vi "FingerTaskHold.vi"() -> ()   [LabVIEW 2011]
doc: "This example is a template that gives the structure of a single-loop PID controller. This VI uses the PID Filter VI to reduce measurement noise. This VI also uses the PID Autotuning VI to tune the controller based on the closed-loop response. This VI also uses the Timed Loop to ensure deterministic execution.\n\nReplace the Dummy Input and Dummy Output VIs with code that communicates with a real-time target."
uses:
  <vilib>/addons/Digital Filter Design/_Objects.llb/DFD Filter Obj.ctl
  <vilib>/addons/Digital Filter Design/_Objects.llb/DFD Filter Coef.ctl
  <vilib>/addons/Digital Filter Design/_Objects.llb/DFD Filter Structure Type Selector.ctl
  <vilib>/addons/Digital Filter Design/_Objects.llb/dfd_Internal Quantization Settings.ctl
  <vilib>/addons/Digital Filter Design/_Objects.llb/dfd_Internal Quantization Srcs.ctl
  <vilib>/addons/Digital Filter Design/_Objects.llb/DFD Coef Norm Type.ctl
  <vilib>/Platform/TimedLoop/XDataNode/timing_clust.ctl
  <vilib>/Platform/TimedLoop/XDataNode/nitl_modes.ctl
  <vilib>/Platform/TimedLoop/XDataNode/wakeup.ctl
  <vilib>/DAQmx/write.llb/DAQmx Write (Counter Frequency 1Chan 1Samp).vi
  <vilib>/DAQmx/write.llb/DAQmx Write (Digital 1D Bool NChan 1Samp 1Line).vi
  <vilib>/DAQmx/read.llb/DAQmx Read (Counter DBL 1Chan 1Samp).vi
  <vilib>/DAQmx/read.llb/DAQmx Read (Analog 1D DBL NChan 1Samp).vi
  <vilib>/addons/control/pid/pid.llb/PID Advanced (DBL Array).vi
  <vilib>/DAQmx/write.llb/DAQmx Write (Analog DBL 1Chan 1Samp).vi
  <vilib>/DAQmx/write.llb/DAQmx Write (Analog 1D DBL NChan 1Samp).vi
  <vilib>/addons/control/pid/pid.llb/PID Derivative Action Buffered (DBL Array).vi
  <vilib>/addons/control/pid/pid.llb/PID Get Advanced Error (DBL Array).vi
  <vilib>/addons/control/pid/pid.llb/PID Integral Action Buffered (DBL Array).vi
  <vilib>/addons/control/pid/pid.llb/PID Resize 1D Array.vi
  <vilib>/addons/control/pid/pid.llb/PID Get Advanced Error (DBL).vi
  <vilib>/DAQmx/create/channels.llb/DAQmx Create Channel (CO-Pulse Generation-Frequency).vi
  <vilib>/DAQmx/configure/timing.llb/DAQmx Timing (Implicit).vi
  <vilib>/DAQmx/miscellaneous.llb/DAQmx Fill In Error Info.vi
  <vilib>/addons/Digital Filter Design/Process.llb/DFD Filtering (PtByPt NChan).vi
  <vilib>/addons/control/pid/pid.llb/PID Parameter Manager (DBL Array).vi
  <vilib>/Platform/TimedLoop/XDataNode/XDataNode.xnode
  <vilib>/Platform/TimedLoop/XDataNode/XDNodeRunTimeDep.lvlib
  <vilib>/addons/Digital Filter Design/NI_DigFilterLicensed.lvlib
  <vilib>/addons/control/pid/NI_PID_pid.lvlib
panel:
  out "LastCount":u64
  out "error out 2":errorcluster
  out "error out":errorcluster
  in  "Timing":T1={"JuiceTime"=1000.0, "AbortTime"=1000.0, "RampTime"=500, "HoldTime"=1000, "ASD"=500}
  in  "RecordsSelection":string(combo)
  in  "Database":T2={"ExperimentDate"=timestamp(3401556199.892892 s since 1904-01-01), "ImplantDate"=timestamp(3401890063 s since 1904-01-01), "CerebusFolder"="", "Experimenter"="Tyler Davis", "PatientNumber"="201102", "DominantHand"="Right", "DeviceType"="uECOG", "DeviceSerial"="CG-64BPX-F419", "DeviceHemisphere"="Right", "DeviceRegion"="Hand", "TaskType"="ArmMovementTask.vi", "TaskComments"="", "RecordingComments"="", "GeneralObservations"=""}
  in  "CerebusConfigFile":path=path "E:/Code/TaskAutomation/ConfigFiles/32ChanRecording2K.mat"
  out "DatabaseUDL":path=path "E:/Data/PatientDatabase.udl"
  out "DataFolder":string
  out "TaskType":string
  out "Recording":bool
  out "StartTime":timestamp
  in  "MaxForce":dbl
  out "Middle":dbl(slide)=4.88375 scale=0.0..6.0
  out "Index":dbl(slide)=4.76025 scale=0.0..6.0
  out "Thumb":dbl(slide)=4.62875 scale=0.0..6.0
  in  "RandForce":bool
  in  "RampGain":dbl[](array[numeric])=[3.0, 3.0, 3.0] caption="Ramp Force"
  out "EncStartPos":cluster{"Index":dbl, "Middle":dbl, "Ring":dbl}={"Index"=3.1270000000000002, "Middle"=3.3110000000000004, "Ring"=3.0875000000000004}
  in  "HoldRange":dbl[](array[numeric])=[1.0, 1.0, 1.0]
  in  "RandFinger":bool=TRUE
  in  "InitialForce":dbl[](array[numeric])=[1.0, 1.0, 1.0] min=-10.0 max=10.0 step=1.0
  out "SlowLoop":bool
  out "SetPtOut":cluster{"[0]":dbl, "[1]":dbl, "[2]":dbl}(graph)={"[0]"=-0.023249999999999993, "[1]"=-0.6442500000000004, "[2]"=0.49950000000000294} caption="Set Point"
  out "LoadCell":cluster{"[0]":dbl, "[1]":dbl, "[2]":dbl}(graph)={"[0]"=-0.06598031273279871, "[1]"=-0.6487244867483078, "[2]"=0.44124715755068283} caption="Force"
  out "LoopPeriod":u64=10
  in  "DesiredPos":dbl[](array[numeric])=[3.0, 3.0, 3.0]
  out "EncPos":cluster{"[0]":dbl, "[1]":dbl, "[2]":dbl}(graph)={"[0]"=4.76025, "[1]"=4.88375, "[2]"=4.62875} caption="Position"
  out "TrialType":i32=1
  out "TrialCount":i32=2
  out "LoopCount":u64=1552
  out "Current State":T3(ring)=enum."Acquire Start"
  out "Finalize":enum16{"Reward", "Cerebus", "Reset"}(ring)
  out "Outcome":string="--"
  in  "Linearity":dbl=1.0 format="%.2f"
  out "PIDGainsOut":T4(array[cluster])=[{"proportional gain (Kc)"=0.4600000000000001, "integral time (Ti, min)"=0.0, "derivative time (Td, min)"=0.0}, {"proportional gain (Kc)"=0.4600000000000001, "integral time (Ti, min)"=0.0, "derivative time (Td, min)"=0.0}, {"proportional gain (Kc)"=0.4600000000000001, "integral time (Ti, min)"=0.0, "derivative time (Td, min)"=0.0}]
  in  "PIDGains":T5={"proportional high (Kc)"=0.5, "integral high (Ti, min)"=0.0, "derivative high (Td, min)"=0.0, "derivative low (Td, min)"=0.0, "integral low (Ti, min)"=0.0, "proportional low (Kc)"=0.1} caption="PID Gains"
  in  "PWMFreq(Hz)":dbl=20000.0 caption="PWM (Hz)" format="%#.6f"
  out "EncMax":dbl[](array[numeric])=[6.508000000000001, 6.507000000000001, 6.469500000000001]
  in  "BndrsCluster":T6={"InwardLimit(%)"=[0.7, 0.7, 0.7], "OutwardLimit(%)"=[0.3, 0.3, 0.3], "SpringCnst"=[5.0, 5.0, 5.0]} caption="Boundaries"
  out "LP_LoadCell":T7={"mSRate_Fs"=500.0, "mSRate_Version"="2.0", "mSRate_Comments"="", "mSRate_OrgCoef"={"type"=enum."IIR Cascaded Second Order Sections Form II Transposed", "gain"=1.0, "coef a (k)"=[-0.36952737735124136, 0.1958157126558331], "coef b (v)"=[0.20657208382614797, 0.41314416765229595, 0.20657208382614797]}, "mSRate_CurCoef"={"type"=enum."IIR Cascaded Second Order Sections Form II Transposed", "gain"=1.0, "coef a (k)"=[-0.36952737735124136, 0.1958157126558331], "coef b (v)"=[0.20657208382614797, 0.41314416765229595, 0.20657208382614797]}, "mSRate_Quantized?"=FALSE, "mSRate_QCoef"={"type"=enum."Undefined", "gain"=1.0, "coef a (k)"=[], "coef b (v)"=[]}, "mSRate_QSettings"=[], "mSRate_Order"=2, "mSRate_Scaling"={"mSRate_ScaleByPowerOf2?"=FALSE, "mSRate_ScaleType"=enum."No Norm"}} {"mSRate_QSettings"."source" items=["Coef a/k"=0, "Coef b/v"=7, "Input"=1, "Output"=2, "Multiplicand"=3, "Product"=4, "Sum"=5, "Delay"=6, "Gain"=8]}
  in  "LP_LoadCell(Hz)":dbl=100.0
  out "MotorDir":bool[](array[boolean])=[TRUE, TRUE, TRUE]
  in  "LoopFreq(Hz)":dbl=500.0 caption="Loop Period (us)"
  out "SetPoint":dbl[](array[numeric])=[1.0, 1.0, 1.0] caption="Set Point" min=-10.0 max=10.0 step=1.0
  out "PWMTaskC":refnum<k21>
  out "PWMTaskB":refnum<k21>
  in  "PIDLimit":dbl=0.5 caption="MaxDutyCycle" min=0.0 max=1.0 step=0.01 format="%.2f"
  out "LoopPeriodPID(s)":dbl=0.002 caption="Loop Period PID (s)" format="%#_10g"
  out "PWMTaskA":refnum<k21>
  out "LoopDuration(us)":i64=965 caption="Actual Loop Period (us)"
  in  "Stop":bool
  out "SlowLoopPID":bool
  # "index"
  # "middle"
  # "thumb"
  # "limits = -10 to 10 lbs"
  # "limits = 0 to 6 in"
  # "all time in ms"
  # "Do not place ';' or '=' in the comment fields"
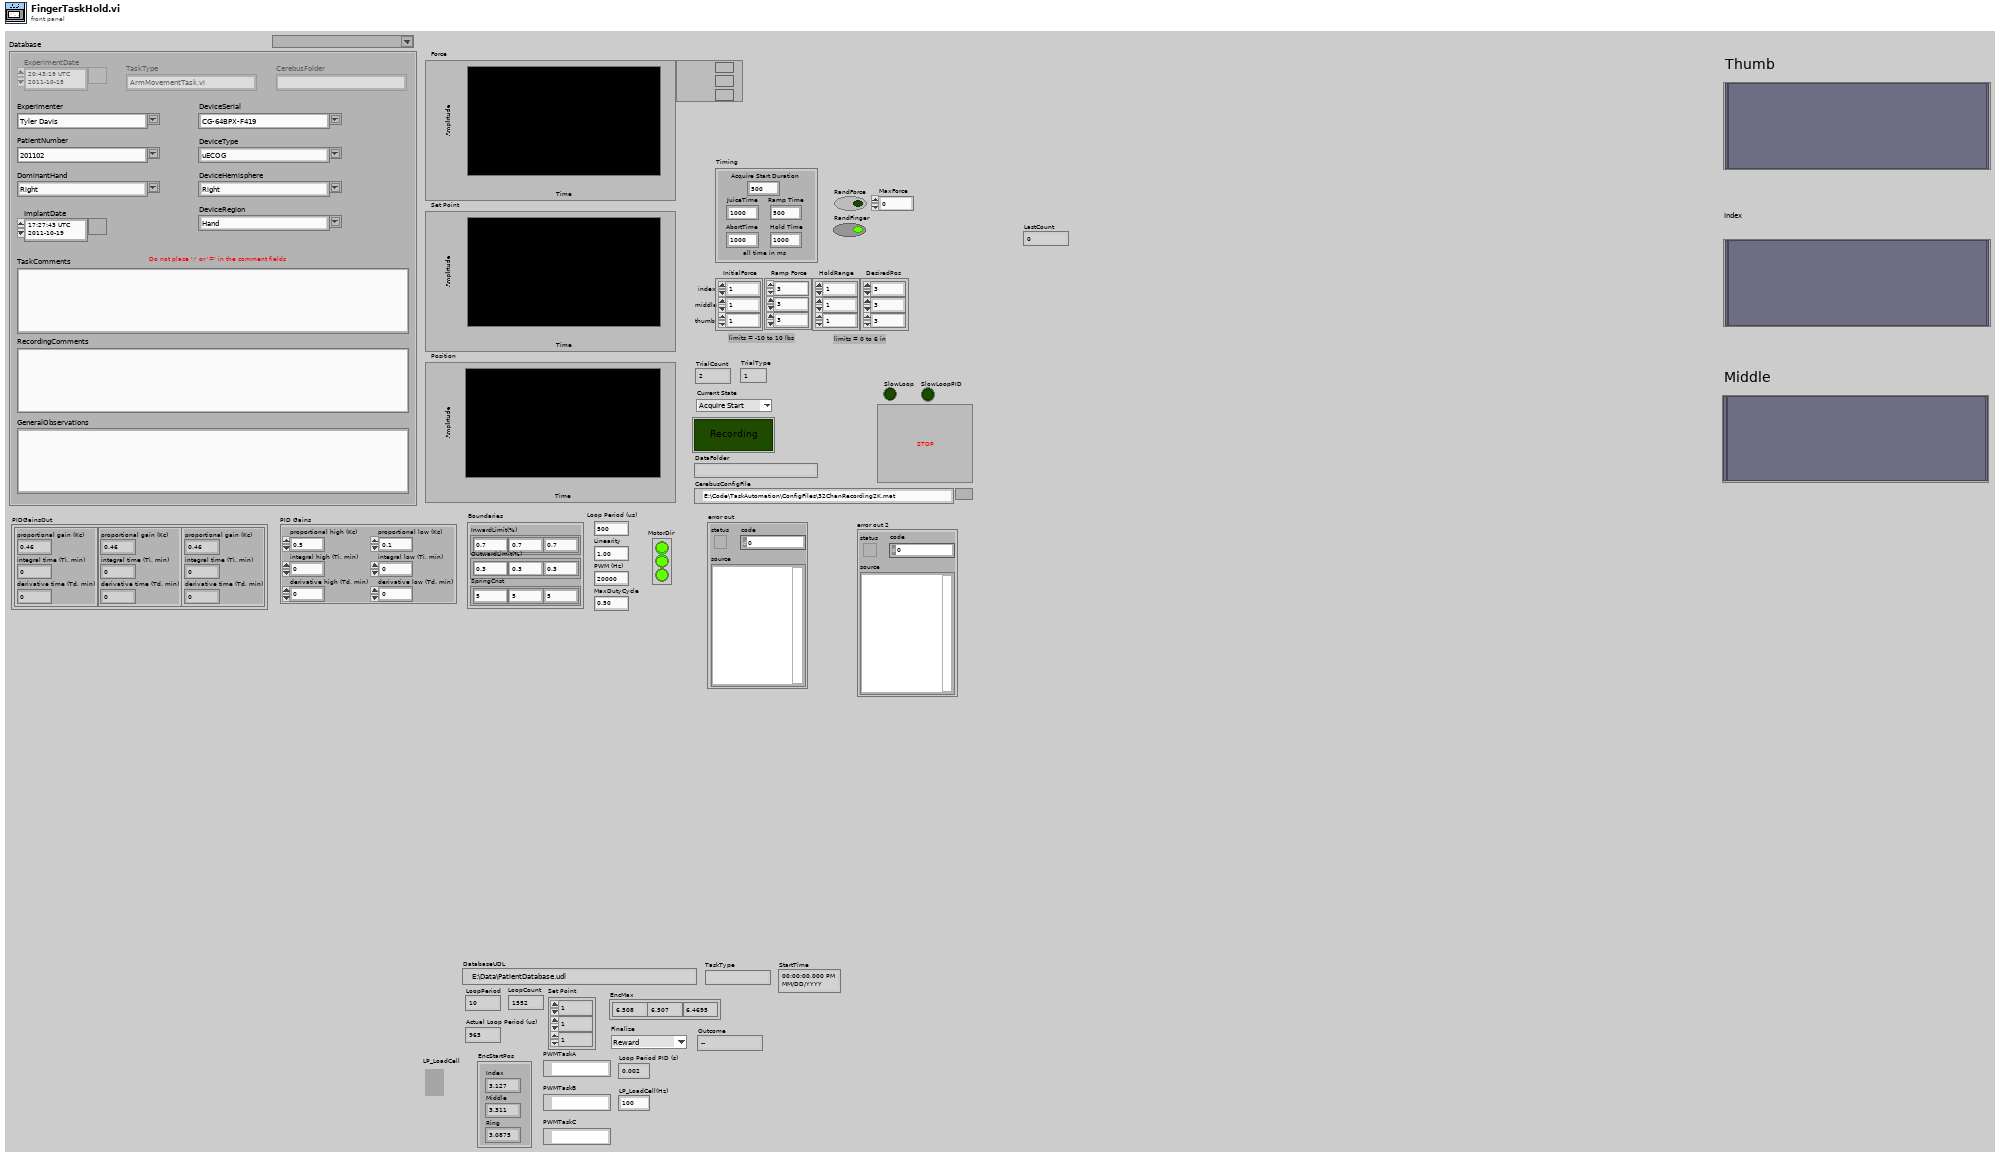
[diagram p1: front panel]
types:
  T1 = cluster{"JuiceTime":dbl, "AbortTime":dbl, "RampTime":u64, "HoldTime":u64, "ASD":u64}
  T2 = cluster{"ExperimentDate":timestamp, "ImplantDate":timestamp, "CerebusFolder":string, "Experimenter":string, "PatientNumber":string, "DominantHand":string, "DeviceType":string, "DeviceSerial":string, "DeviceHemisphere":string, "DeviceRegion":string, "TaskType":string, "TaskComments":string, "RecordingComments":string, "GeneralObservations":string}
  T3 = enum16{"Initialize", "Acquire Start", "Acquire Response", "Finalize"}
  T4 = cluster{"proportional gain (Kc)":dbl, "integral time (Ti, min)":dbl, "derivative time (Td, min)":dbl}[]
  T5 = cluster{"proportional high (Kc)":dbl, "integral high (Ti, min)":dbl, "derivative high (Td, min)":dbl, "derivative low (Td, min)":dbl, "integral low (Ti, min)":dbl, "proportional low (Kc)":dbl}
  T6 = cluster{"InwardLimit(%)":dbl[], "OutwardLimit(%)":dbl[], "SpringCnst":dbl[]}
  T7 = typedef "NI_DigFilterLicensed.lvlib/DFD Filter Obj.ctl" = cluster{"mSRate_Fs":dbl, "mSRate_Version":string, "mSRate_Comments":string, "mSRate_OrgCoef":T8, "mSRate_CurCoef":T8, "mSRate_Quantized?":bool, "mSRate_QCoef":T8, "mSRate_QSettings":T10[], "mSRate_Order":i32, "mSRate_Scaling":cluster{"mSRate_ScaleByPowerOf2?":bool, "mSRate_ScaleType":T12}}
  T8 = typedef "NI_DigFilterLicensed.lvlib/DFD Filter Coef.ctl" = cluster{"type":T9, "gain":dbl, "coef a (k)":dbl[], "coef b (v)":dbl[]}
  T9 = typedef "NI_DigFilterLicensed.lvlib/DFD Filter Structure Type Selector.ctl" = enum16{"Undefined", "FIR Direct Form", "FIR Direct Form Transposed", "FIR Symmetric", "FIR Antisymmetric", "IIR Direct Form I", "IIR Direct Form I Transposed", "IIR Direct Form II", "IIR Direct Form II Transposed", "IIR Cascaded Second Order Sections Form I", "IIR Cascaded Second Order Sections Form I Transposed", "IIR Cascaded Second Order Sections Form II", "IIR Cascaded Second Order Sections Form II Transposed", "Lattice Allpass (basic sections)", "Lattice Allpass (one multiplier sections)", "Lattice Allpass (normalized sections)", "Lattice AR (basic sections)", "Lattice AR (one multiplier sections)", "Lattice AR (normalized sections)", "Lattice MA (minimum phase)", "Lattice MA (maximum phase)", "Lattice ARMA (basic sections)", "Lattice ARMA (one multiplier sections)", "Lattice ARMA (normalized sections)"}
  T10 = typedef "NI_DigFilterLicensed.lvlib/dfd_Internal Quantization Settings.ctl" = cluster{"source":T11, "wl":i16, "iwl":i16, "overflow mode":enum16{"Saturation", "Wrap"}, "rounding mode":enum16{"Nearest", "Truncation"}, "signed?":bool}
  T11 = typedef "NI_DigFilterLicensed.lvlib/dfd_Internal Quantization Srcs.ctl" = u16
  T12 = typedef "NI_DigFilterLicensed.lvlib/DFD Coef Norm Type.ctl" = enum16{"No Norm", "Time Domain 1-Norm", "Time Domain 2-Norm", "Time Domain Inf-Norm"}
  T13 = enum16{"Initialize", "String", "Start", "New Session", "Stop", "Resume", "Close"}
  T14 = enum16{"SaveConfiguration", "StartRecording", "StopRecording"}
  T15 = typedef "XDNodeRunTimeDep.lvlib/timing_clust.ctl" = cluster{"Expected End [f-1]":u64, "Actual End [f-1]":u64, "Finished Late? [f-1]":bool, "Expected End [i-1]":u64, "Actual End [i-1]":u64, "Finished Late? [i-1]":bool, "Expected Start [i]":u64, "Actual Start [i]":u64, "Expected Start [f]":u64, "Actual Start [f]":u64, "Source Name":string, "Structure Name":string, "Period":i64, "Deadline":i64, "Offset":i64, "Start":i64, "Priority":i32, "Timeout":i32, "Mode":T16, "Wakeup Reason":T17, "Error":errorcluster, "Source Type":string, "Secondary Source Type":string, "Global End Time":u64, "Global Start Time":u64, "Frame Duration":u64, "Iteration Duration":u64, "Assigned CPU":i32, "I/O Scan Engine Mode":u32}
  T16 = typedef "XDNodeRunTimeDep.lvlib/nitl_modes.ctl" = enum32{"No Change", "Process missed periods, maintain original phase", "Discard missed periods, maintain original phase", "Process missed periods, ignore original phase", "Discard missed periods, ignore original phase"}
  T17 = typedef "XDNodeRunTimeDep.lvlib/wakeup.ctl" = enum32{"Normal", "Aborted", "Asynchronous wakeup", "Timing source error", "Timed loop error", "Timeout"}
  T18 = enum16{"Lowpass", "Highpass", "Bandpass", "Bandstop"}
  T19 = typedef "LVAllMonitorsDisplayTypeDef.ctl" = cluster{"Bounds":cluster{"Left":i16, "Top":i16, "Right":i16, "Bottom":i16}, "Depth":i16}[]
  T20 = cluster{"Disp.AllMonitors[0]":cluster{"Bounds":cluster{"Left":i16, "Top":i16, "Right":i16, "Bottom":i16}, "Depth":i16}, "Disp.AllMonitors[1]":cluster{"Bounds":cluster{"Left":i16, "Top":i16, "Right":i16, "Bottom":i16}, "Depth":i16}, "Disp.AllMonitors[2]":cluster{"Bounds":cluster{"Left":i16, "Top":i16, "Right":i16, "Bottom":i16}, "Depth":i16}, "Disp.AllMonitors[3]":cluster{"Bounds":cluster{"Left":i16, "Top":i16, "Right":i16, "Bottom":i16}, "Depth":i16}, "Disp.AllMonitors[4]":cluster{"Bounds":cluster{"Left":i16, "Top":i16, "Right":i16, "Bottom":i16}, "Depth":i16}, "Disp.AllMonitors[5]":cluster{"Bounds":cluster{"Left":i16, "Top":i16, "Right":i16, "Bottom":i16}, "Depth":i16}, "Disp.AllMonitors[6]":cluster{"Bounds":cluster{"Left":i16, "Top":i16, "Right":i16, "Bottom":i16}, "Depth":i16}, "Disp.AllMonitors[7]":cluster{"Bounds":cluster{"Left":i16, "Top":i16, "Right":i16, "Bottom":i16}, "Depth":i16}, "Disp.AllMonitors[8]":cluster{"Bounds":cluster{"Left":i16, "Top":i16, "Right":i16, "Bottom":i16}, "Depth":i16}}
  T21 = cluster{"Left":i16, "Top":i16, "Right":i16, "Bottom":i16}
  T22 = cluster{"Left":bool, "Top":bool, "Right":bool, "Bottom":bool}
  T23 = typedef "LVRectTypeDef.ctl" = cluster{"left":i16, "top":i16, "right":i16, "bottom":i16}
  T24 = typedef "LVPointTypeDef.ctl" = cluster{"Horizontal":i16, "Vertical":i16}
  T25 = cluster{"SetPointOut[0]":dbl, "SetPointOut[1]":dbl, "SetPointOut[2]":dbl}
  T26 = cluster{"signal out[0]":dbl, "signal out[1]":dbl, "signal out[2]":dbl}
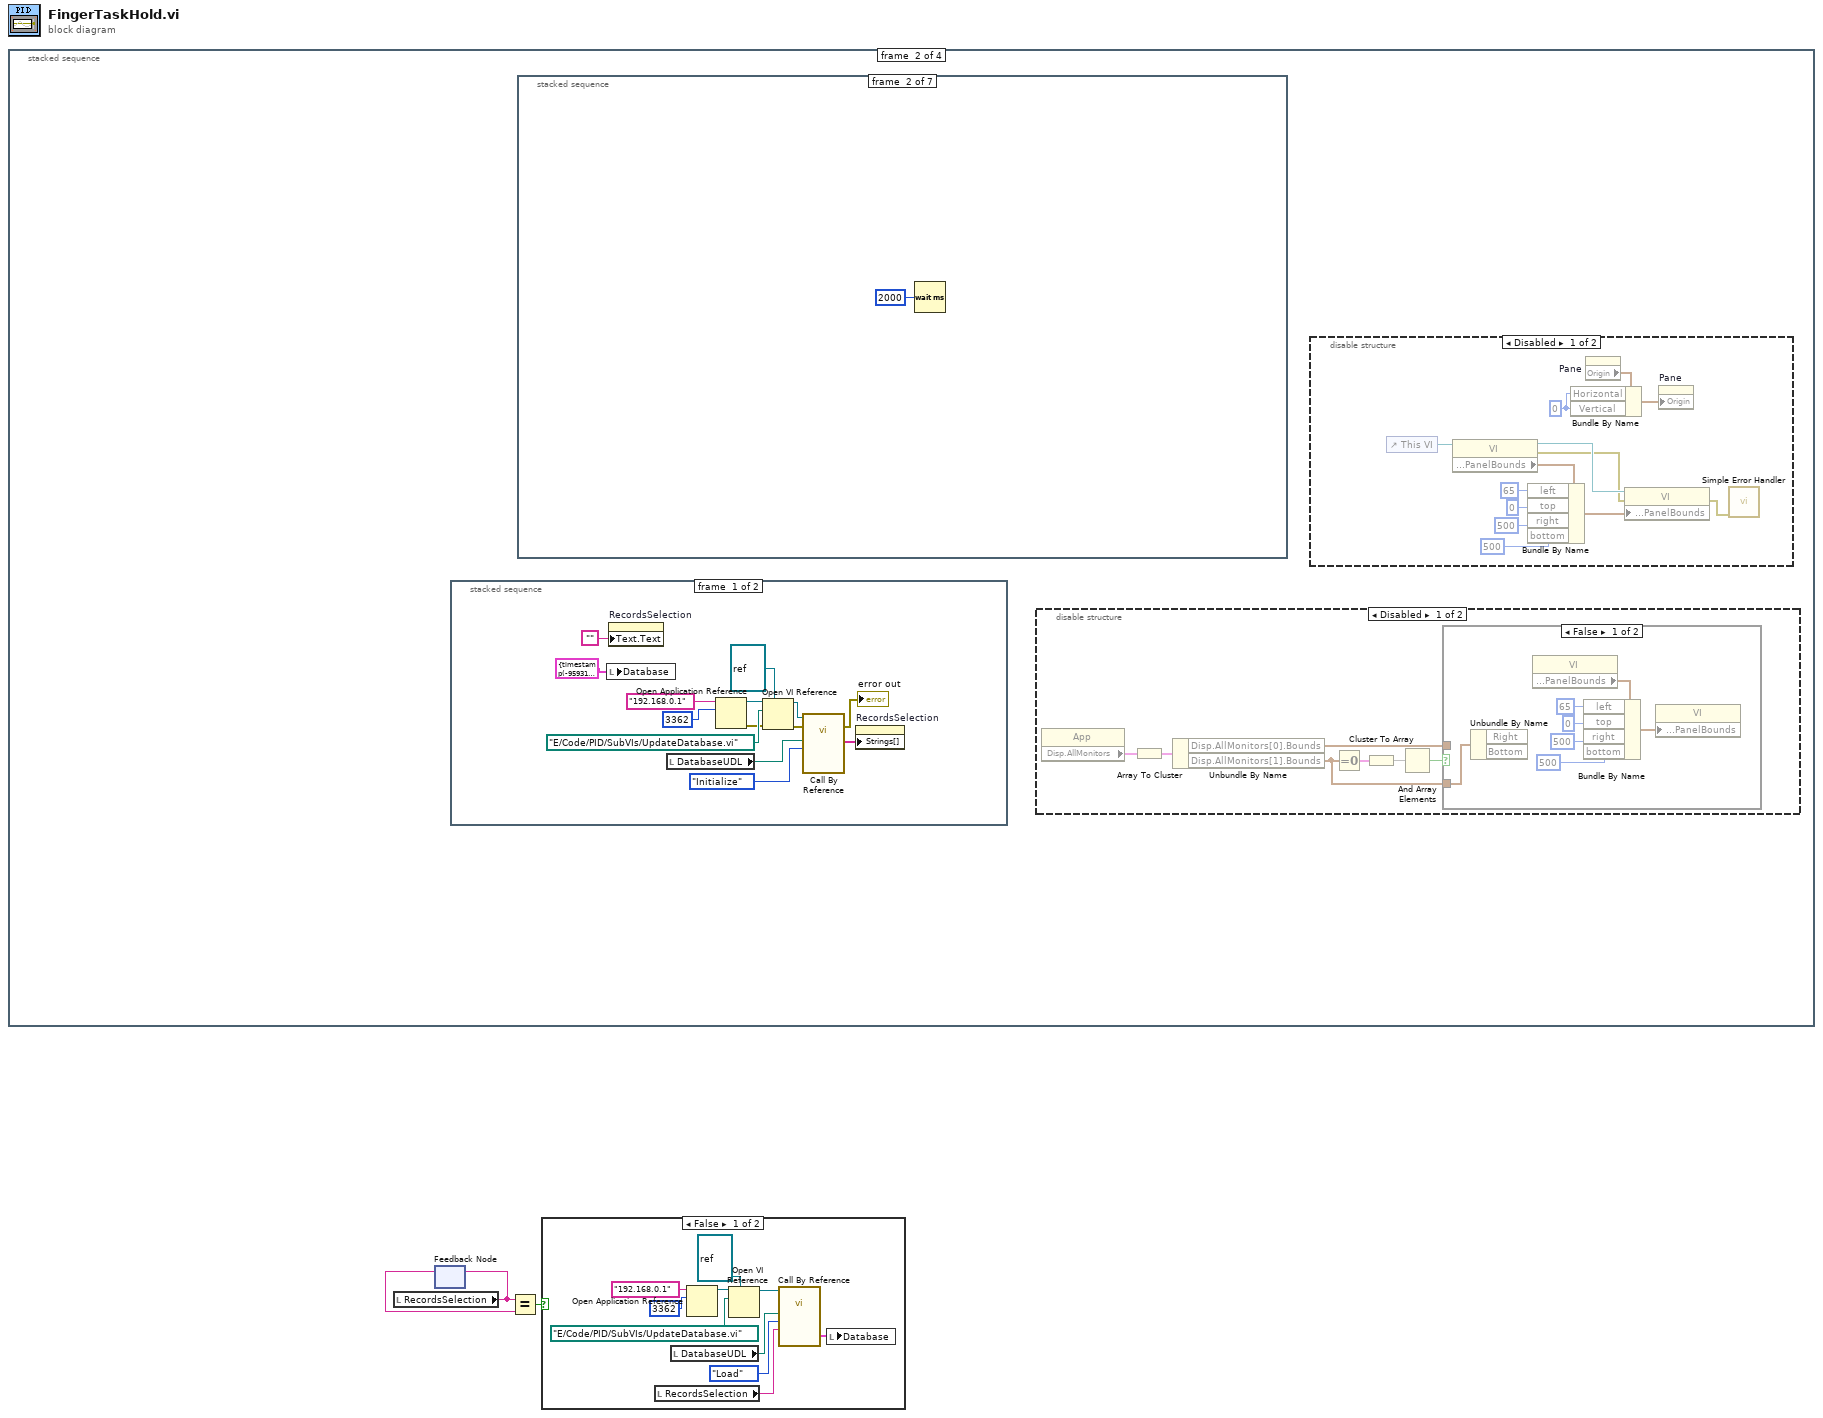
[diagram p0: block diagram]
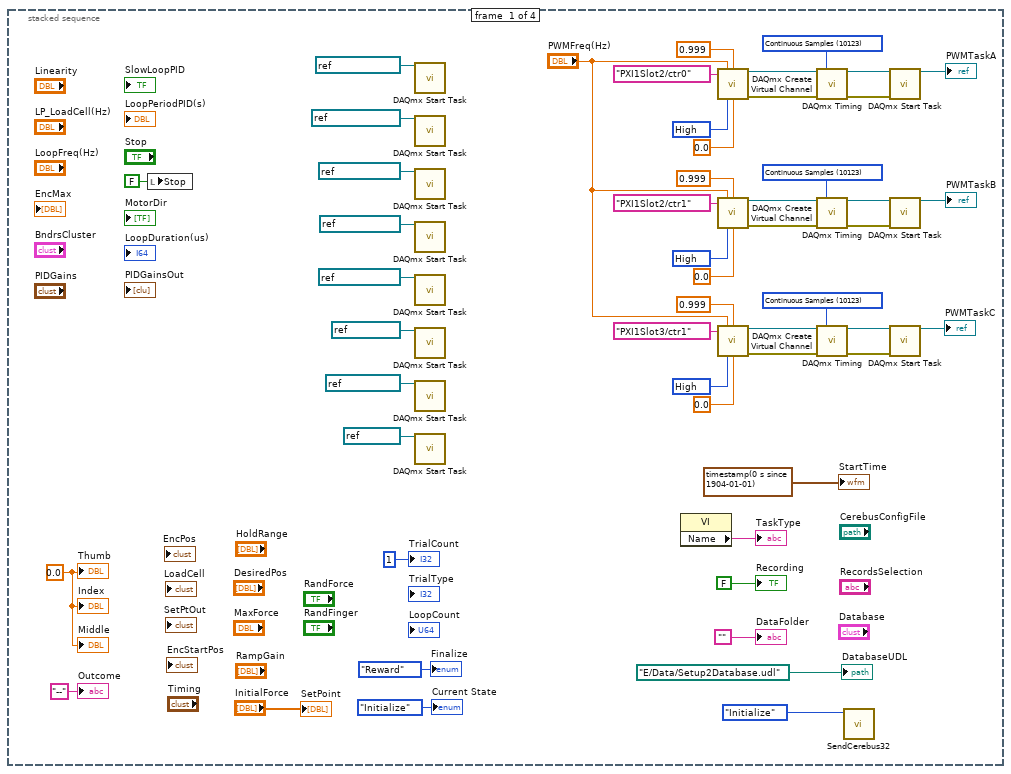
[diagram p3: hidden frame]
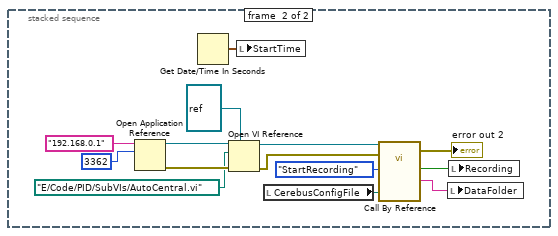
[diagram p4: hidden frame]
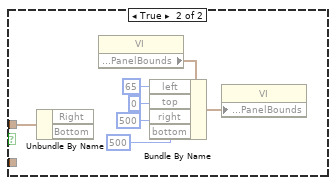
[diagram p6: hidden frame]
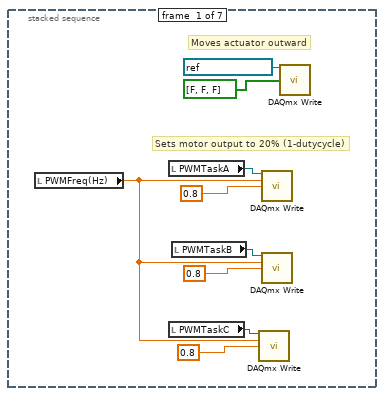
[diagram p8: hidden frame]
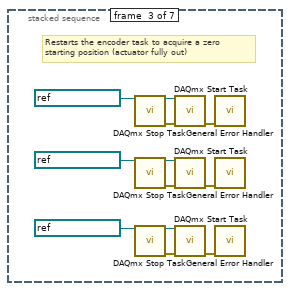
[diagram p9: hidden frame]
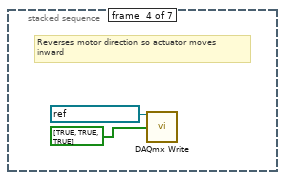
[diagram p10: hidden frame]
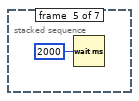
[diagram p11: hidden frame]
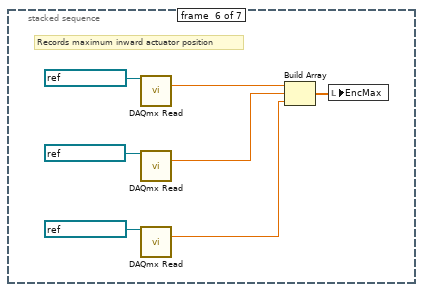
[diagram p12: hidden frame]
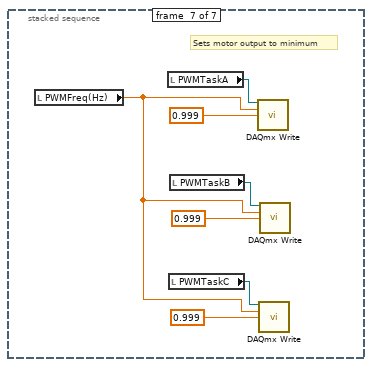
[diagram p13: hidden frame]
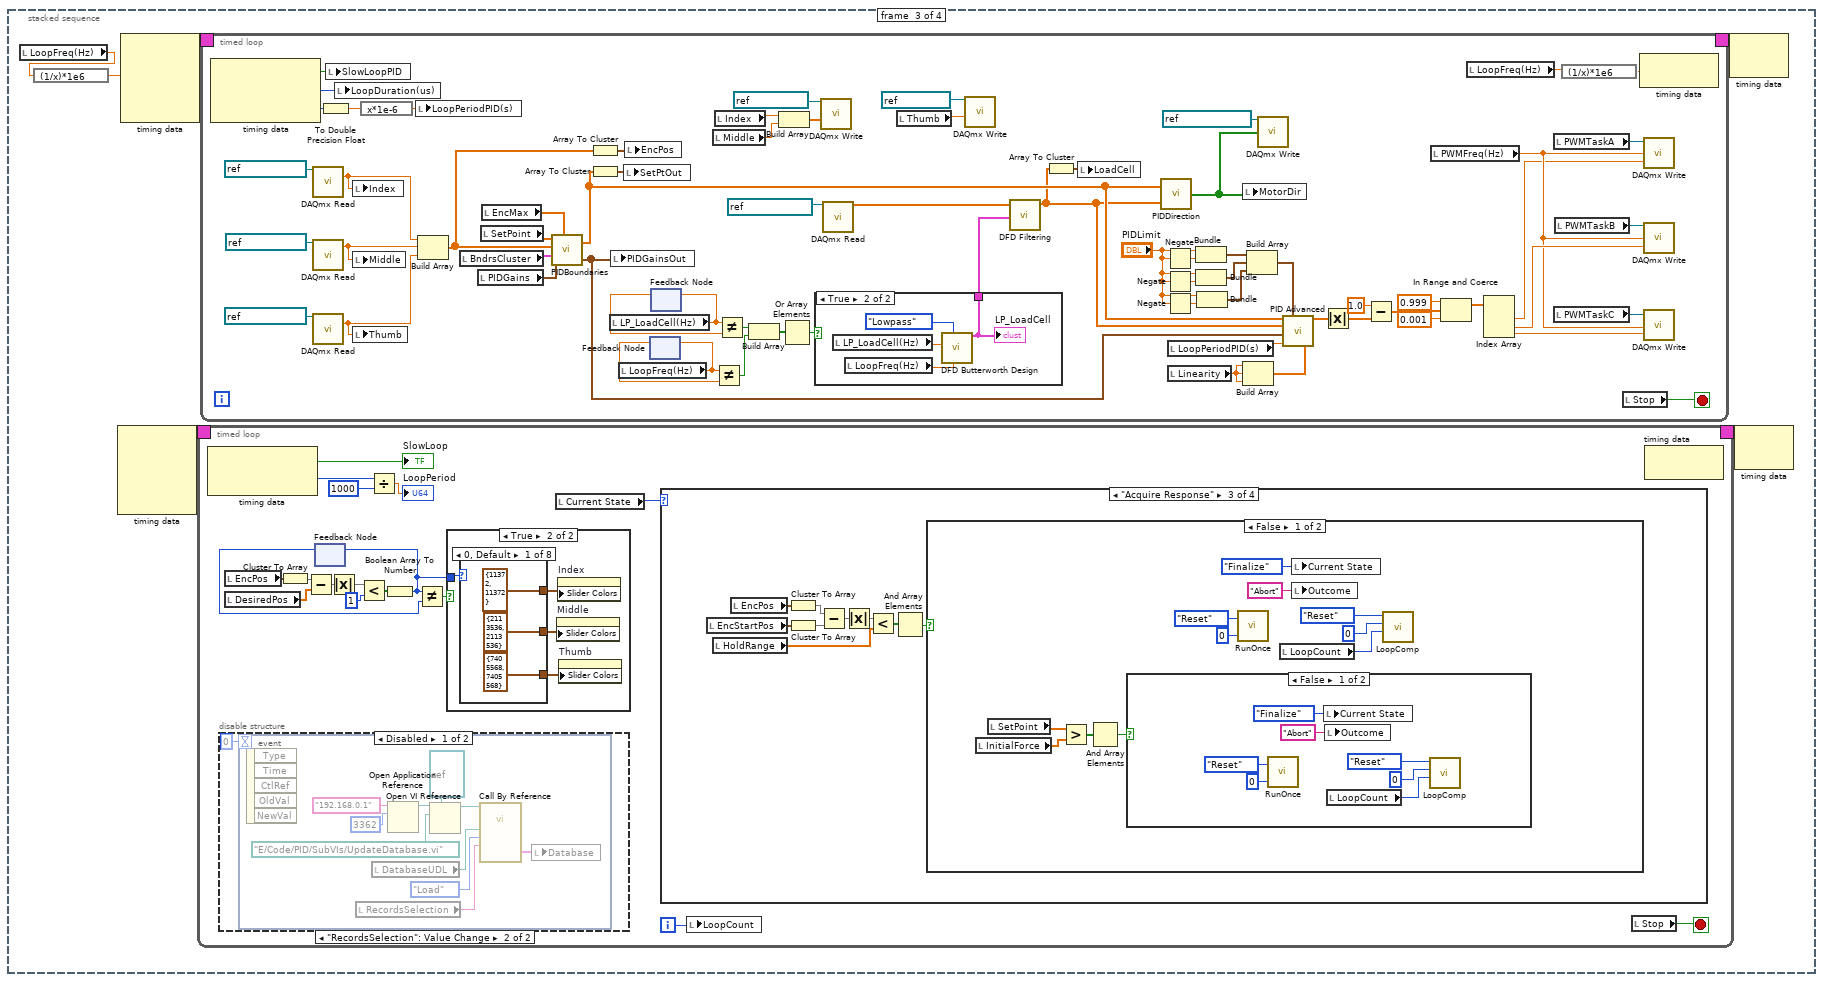
[diagram p14: hidden frame]
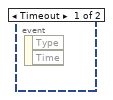
[diagram p15: hidden frame]
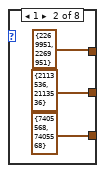
[diagram p18: hidden frame]
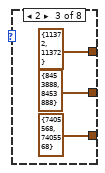
[diagram p19: hidden frame]
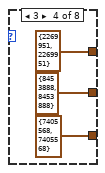
[diagram p20: hidden frame]
diagram:
  n1 = stacked-sequence {
    frame #0 {
      w11 = 0.0 ("THUMB")
      w28 = 10192 items=["High"=10192, "Low"=10214] ("idle state")
      w22 = 10123 items=["Finite Samples"=10178, "Continuous Samples"=10123] ("sample mode")
      w35 = 10192 items=["High"=10192, "Low"=10214] ("idle state")
      w41 = 10123 items=["Finite Samples"=10178, "Continuous Samples"=10123] ("sample mode")
      w52 = 10192 items=["High"=10192, "Low"=10214] ("idle state")
      w45 = 10123 items=["Finite Samples"=10178, "Continuous Samples"=10123] ("sample mode")
      n2 = local write "Stop"(FALSE ("stop")) -> ()
      n3 = call <vilib>:"DAQmx Start Task.vi"("task/channels in"=refnum<k21> "ForceInABC") -> ()  [unwired: 13 in, 2 out]
      n4 = call <vilib>:"DAQmx Start Task.vi"("task/channels in"=refnum<k21> "MotorDirABC") -> ()  [unwired: 13 in, 2 out]
      n5 = call <vilib>:"DAQmx Start Task.vi"("task/channels in"=refnum<k21> "PositionInA") -> ()  [unwired: 13 in, 2 out]
      n6 = call <vilib>:"DAQmx Start Task.vi"("task/channels in"=refnum<k21> "PositionInB" ("task")) -> ()  [unwired: 13 in, 2 out]
      n7 = call <vilib>:"DAQmx Start Task.vi"("task/channels in"=refnum<k21> "PositionInC") -> ()  [unwired: 13 in, 2 out]
      n8 = call <vilib>:"DAQmx Start Task.vi"("task/channels in"=refnum<k21> "PosOutT" ("task")) -> ()  [unwired: 13 in, 2 out]
      n9 = call <vilib>:"DAQmx Start Task.vi"("task/channels in"=refnum<k21> "PosOutIM") -> ()  [unwired: 13 in, 2 out]
      n10 = call <vilib>:"DAQmx Start Task.vi"("task/channels in"=refnum<k21> "sound") -> ()  [unwired: 13 in, 2 out]
      n11 = property class="VI"() -> ("Name"=→"TaskType":string)  [unwired: 2 in, 2 out]
      n12 = call-poly <vilib>:"DAQmx Create Virtual Channel.vi"("frequency"="PWMFreq(Hz)", "duty cycle"=0.999, "counter"=tag "PXI1Slot2/ctr0", "idle state"=w52, "initial delay"=0.0) -> ("task out"=w48:refnum<k21>, "error out"=w49:errorcluster)  [unwired: 9 in]
      n13 = call-poly <vilib>:"DAQmx Create Virtual Channel.vi"("frequency"="PWMFreq(Hz)", "duty cycle"=0.999, "counter"=tag "PXI1Slot2/ctr1", "idle state"=w35, "initial delay"=0.0) -> ("task out"=w38:refnum<k21>, "error out"=w37:errorcluster)  [unwired: 9 in]
      n14 = call-poly <vilib>:"DAQmx Create Virtual Channel.vi"("frequency"="PWMFreq(Hz)", "duty cycle"=0.999, "counter"=tag "PXI1Slot3/ctr1", "idle state"=w28, "initial delay"=0.0) -> ("task out"=w25:refnum<k21>, "error out"=w26:errorcluster)  [unwired: 9 in]
      n15 = call-poly <vilib>:"DAQmx Timing.vi"("task/channels in"=w48, "sample mode"=w45, "error in"=w49) -> ("task out"=w46:refnum<k21>, "error out"=w47:errorcluster)  [unwired: 11 in]
      n16 = call-poly <vilib>:"DAQmx Timing.vi"("task/channels in"=w38, "sample mode"=w41, "error in"=w37) -> ("task out"=w40:refnum<k21>, "error out"=w39:errorcluster)  [unwired: 11 in]
      n17 = call-poly <vilib>:"DAQmx Timing.vi"("task/channels in"=w25, "sample mode"=w22, "error in"=w26) -> ("task out"=w23:refnum<k21>, "error out"=w24:errorcluster)  [unwired: 11 in]
      n18 = call "SendCerebus32.vi"("Mode"=T13."Initialize") -> ()  [unwired: 4 in]
      n19 = call <vilib>:"DAQmx Start Task.vi"("task/channels in"=w46, "error in"=w47) -> ("task out"=→"PWMTaskA":refnum<k21>)  [unwired: 12 in, 1 out]
      n20 = call <vilib>:"DAQmx Start Task.vi"("task/channels in"=w40, "error in"=w39) -> ("task out"=→"PWMTaskB":refnum<k21>)  [unwired: 12 in, 1 out]
      n21 = call <vilib>:"DAQmx Start Task.vi"("task/channels in"=w23, "error in"=w24) -> ("task out"=→"PWMTaskC":refnum<k21>)  [unwired: 12 in, 1 out]
      "SetPoint" <- "InitialForce"
      "Outcome" <- "--" ("Outcome")
      "Current State" <- T3."Initialize" ("Current State")
      "Finalize" <- enum16{"Reward", "Cerebus", "Reset"}."Reward" ("Finalize")
      "TrialCount" <- 1 ("TrialCount")
      "Thumb" <- w11
      "Index" <- w11
      "Middle" <- w11
      "StartTime" <- timestamp(0 s since 1904-01-01)
      "Recording" <- FALSE ("Recording")
      "DatabaseUDL" <- path "E:/Data/Setup2Database.udl" ("DatabaseUDL")
      "DataFolder" <- ""
    }
    frame #1 {
      n22 = stacked-sequence {
        frame #0 {
          n23 = local write "Database"(T2 {"ExperimentDate"=timestamp(-9593179200 s since 1904-01-01), "ImplantDate"=timestamp(-9593179200 s since 1904-01-01), "CerebusFolder"="", "Experimenter"="", "PatientNumber"="", "DominantHand"="", "DeviceType"="", "DeviceSerial"="", "DeviceHemisphere"="", "DeviceRegion"="", "TaskType"="", "TaskComments"="", "RecordingComments"="", "GeneralObservations"=""} ("Database")) -> ()
          n24 = property on="RecordsSelection" class="CmbBox"("Text.Text"="") -> ()  [unwired: 2 in, 2 out]
          n25 = local read "DatabaseUDL"() -> (w60:path)
          n26 = Open Application Reference(10:u16 3362 ("port number or service name (3363)"), 11:"192.168.0.1" ("machine name (\"\":  open local reference)")) -> (0:w58:errorcluster, 3:w65:refnum<vi>)  [unwired: 2 in]
          n27 = Open VI Reference(type specifier VI Refnum (for type only)=refnum<vi> refnum, application reference (local)=w65, vi path=path "E:/Code/PID/SubVIs/UpdateDatabase.vi", error in (no error)=w58) -> (vi reference=w62:refnum<vi>, error out=w57:errorcluster)  [unwired: 2 in]
          n28 = call-by-ref "?"(reference=w62, error in=w57, "CallType"=enum16{"Initialize", "Save", "Load"}."Initialize", "DatabaseUDL"=w60) -> (error out=→"error out":errorcluster, "ExperimentDatesSorted"=w59:string[])  [unwired: 2 in, 3 out]
          n29 = property on="RecordsSelection" class="CmbBox"("Strings[]"=w59) -> ()  [unwired: 2 in, 2 out]
        }
        frame #1 {
          n30 = Open Application Reference(10:u16 3362 ("port number or service name (3363)"), 11:"192.168.0.1" ("machine name (\"\":  open local reference)")) -> (0:w73:errorcluster, 3:w80:refnum<vi>)  [unwired: 2 in]
          n31 = Get Date/Time In Seconds() -> (seconds since 1Jan1904=w83:timestamp)
          n32 = Open VI Reference(type specifier VI Refnum (for type only)=refnum<vi> refnum, application reference (local)=w80, vi path=path "E:/Code/PID/SubVIs/AutoCentral.vi", error in (no error)=w73) -> (vi reference=w78:refnum<vi>, error out=w72:errorcluster)  [unwired: 2 in]
          n33 = local write "StartTime"(w83) -> ()
          n34 = local read "CerebusConfigFile"() -> (w76:path)
          n35 = call-by-ref "?"(reference=w78, error in=w72, "ConfigurationFile"=w76, "Mode"=T14."StartRecording") -> (error out=→"error out 2":errorcluster, "DataFolder"=w74:string, "Recording?"=w75:bool)  [unwired: 1 in, 2 out]
          n36 = local write "DataFolder"(w74) -> ()
          n37 = local write "Recording"(w75) -> ()
        }
      }
      n38 = stacked-sequence {
        frame #0 {
          # "Sets motor output to 20% (1-dutycycle)"
          # "Moves actuator outward"
          n39 = local read "PWMFreq(Hz)"() -> (w118:dbl)
          n40 = local read "PWMTaskA"() -> (w125:refnum<k21>)
          n41 = local read "PWMTaskC"() -> (w119:refnum<k21>)
          n42 = local read "PWMTaskB"() -> (w122:refnum<k21>)
          n43 = call-poly <vilib>:"DAQmx Write.vi"("task/channels in"=w119, "frequency"=w118, "duty cycle"=0.8) -> ()  [unwired: 10 in, 3 out]
          n44 = call-poly <vilib>:"DAQmx Write.vi"("task/channels in"=w125, "frequency"=w118, "duty cycle"=0.8) -> ()  [unwired: 10 in, 3 out]
          n45 = call-poly <vilib>:"DAQmx Write.vi"("task/channels in"=w122, "frequency"=w118, "duty cycle"=0.8) -> ()  [unwired: 10 in, 3 out]
          n46 = call-poly <vilib>:"DAQmx Write.vi"("task/channels in"=refnum<k21> "MotorDirABC", "data"=bool[] [FALSE, FALSE, FALSE]) -> ()  [unwired: 11 in, 3 out]
        }
        frame #1 {
          n47 = Wait (ms)(milliseconds to wait=u32 2000) -> ()  [unwired: 1 out]
        }
        frame #2 {
          # "Restarts the encoder task to acquire a zero\nstarting position (actuator fully out)"
          n48 = call <vilib>:"DAQmx Stop Task.vi"("task/channels in"=refnum<k21> "PositionInA") -> ("task out"=w137:refnum<k21>, "error out"=w136:errorcluster)  [unwired: 13 in]
          n49 = call <vilib>:"DAQmx Stop Task.vi"("task/channels in"=refnum<k21> "PositionInB") -> ("task out"=w134:refnum<k21>, "error out"=w135:errorcluster)  [unwired: 13 in]
          n50 = call <vilib>:"DAQmx Stop Task.vi"("task/channels in"=refnum<k21> "PositionInC") -> ("task out"=w129:refnum<k21>, "error out"=w128:errorcluster)  [unwired: 13 in]
          n51 = call <vilib>:"DAQmx Start Task.vi"("task/channels in"=w137, "error in"=w136) -> ("error out"=w139:errorcluster)  [unwired: 12 in, 1 out]
          n52 = call <vilib>:"DAQmx Start Task.vi"("task/channels in"=w134, "error in"=w135) -> ("error out"=w132:errorcluster)  [unwired: 12 in, 1 out]
          n53 = call <vilib>:"DAQmx Start Task.vi"("task/channels in"=w129, "error in"=w128) -> ("error out"=w131:errorcluster)  [unwired: 12 in, 1 out]
          n54 = call <vilib>:"General Error Handler.vi"("error in (no error)"=w139) -> ()  [unwired: 10 in, 5 out]
          n55 = call <vilib>:"General Error Handler.vi"("error in (no error)"=w132) -> ()  [unwired: 10 in, 5 out]
          n56 = call <vilib>:"General Error Handler.vi"("error in (no error)"=w131) -> ()  [unwired: 10 in, 5 out]
        }
        frame #3 {
          # "Reverses motor direction so actuator moves\ninward"
          n57 = call-poly <vilib>:"DAQmx Write.vi"("task/channels in"=refnum<k21> "MotorDirABC", "data"=bool[] [TRUE, TRUE, TRUE]) -> ()  [unwired: 11 in, 3 out]
        }
        frame #4 {
          n58 = Wait (ms)(milliseconds to wait=u32 2000) -> ()  [unwired: 1 out]
        }
        frame #5 {
          # "Records maximum inward actuator position"
          n59 = call-poly <vilib>:"DAQmx Read.vi"("task/channels in"=refnum<k21> "PositionInA") -> ("data"=w146:dbl)  [unwired: 12 in, 2 out]
          n60 = call-poly <vilib>:"DAQmx Read.vi"("task/channels in"=refnum<k21> "PositionInB") -> ("data"=w145:dbl)  [unwired: 12 in, 2 out]
          n61 = call-poly <vilib>:"DAQmx Read.vi"("task/channels in"=refnum<k21> "PositionInC") -> ("data"=w144:dbl)  [unwired: 12 in, 2 out]
          n62 = Build Array(w146, w145, w144) -> (w143:dbl[])
          n63 = local write "EncMax"(w143) -> ()
        }
        frame #6 {
          # "Sets motor output to minimum"
          n64 = local read "PWMFreq(Hz)"() -> (w150:dbl)
          n65 = local read "PWMTaskA"() -> (w155:refnum<k21>)
          n66 = local read "PWMTaskC"() -> (w151:refnum<k21>)
          n67 = local read "PWMTaskB"() -> (w154:refnum<k21>)
          n68 = call-poly <vilib>:"DAQmx Write.vi"("task/channels in"=w155, "frequency"=w150, "duty cycle"=0.999) -> ()  [unwired: 10 in, 3 out]
          n69 = call-poly <vilib>:"DAQmx Write.vi"("task/channels in"=w151, "frequency"=w150, "duty cycle"=0.999) -> ()  [unwired: 10 in, 3 out]
          n70 = call-poly <vilib>:"DAQmx Write.vi"("task/channels in"=w154, "frequency"=w150, "duty cycle"=0.999) -> ()  [unwired: 10 in, 3 out]
        }
      }
      n71 = disable-structure shown="Disabled" {
        frame Disabled {
          n72 = property class="App"() -> ("Disp.AllMonitors"=w97:T19)  [unwired: 2 in, 2 out]
          n73 = Array To Cluster(array=w97) -> (cluster=w98:T20)
          n74 = Unbundle By Name(w98) -> ("Disp.AllMonitors[0].Bounds"=w102:T21, "Disp.AllMonitors[1].Bounds"=w103:T21)
          n75 = Equal To 0?(x=w103) -> (x = 0?=w99:T22)
          n76 = Cluster To Array(cluster=w99) -> (array=w100:bool[])
          n77 = And Array Elements(Boolean array=w100) -> (logical AND=w101:bool)
          n78 = case shown="False" w101 {
            tunnel: w102 -> [_ w113]
            tunnel: w103 -> [w106 _]
            frame False {
              n79 = Unbundle By Name(w106) -> ()  [unwired: 2 out]
              n80 = property class="VI"() -> ("Front Panel.PanelBounds"=w107:T23)  [unwired: 2 in, 2 out]
              n81 = Bundle By Name(cluster=w107, "left"=i16 65, "top"=i16 0, "right"=i16 500, "bottom"=i16 500) -> (w108:T23)
              n82 = property class="VI"("Front Panel.PanelBounds"=w108) -> ()  [unwired: 2 in, 2 out]
            }
            frame True {
              n83 = Unbundle By Name(w113) -> ()  [unwired: 2 out]
              n84 = property class="VI"() -> ("Front Panel.PanelBounds"=w114:T23)  [unwired: 2 in, 2 out]
              n85 = Bundle By Name(cluster=w114, "left"=i16 65, "top"=i16 0, "right"=i16 500, "bottom"=i16 500) -> (w115:T23)
              n86 = property class="VI"("Front Panel.PanelBounds"=w115) -> ()  [unwired: 2 in, 2 out]
            }
          }
        }
        frame Enabled {
        }
      }
      n87 = disable-structure shown="Disabled" {
        frame Disabled {
          w96 = i16 0 ("Vertical")
          n88 = control-ref of="This VI"() -> (w85:refnum<vi>)
          n89 = property class="VI"(reference=w85) -> (reference out=w87:refnum<vi>, error out=w84:errorcluster, "Front Panel.PanelBounds"=w91:T23)  [unwired: 1 in]
          n90 = Bundle By Name(cluster=w91, "left"=i16 65, "top"=i16 0, "right"=i16 500, "bottom"=i16 500) -> (w90:T23)
          n91 = property on="Pane" class="Pane"() -> ("Origin"=w95:T24)  [unwired: 2 in, 2 out]
          n92 = Bundle By Name(cluster=w95, "Horizontal"=w96, "Vertical"=w96) -> (w94:T24)
          n93 = property class="VI"(reference=w87, error in=w84, "Front Panel.PanelBounds"=w90) -> (error out=w86:errorcluster)  [unwired: 1 out]
          n94 = property on="Pane" class="Pane"("Origin"=w94) -> ()  [unwired: 2 in, 2 out]
          n95 = call <vilib>:"Simple Error Handler.vi"("error in (no error)"=w86) -> ()  [unwired: 4 in, 5 out]
        }
        frame Enabled {
        }
      }
    }
    frame #2 {
      n96 = local read "LoopFreq(Hz)"() -> (w157:dbl)
      n97 = expression code="(1/x)*1e6"(w157) -> (w160:dbl)
      n98 = node-c288() -> (w159:T15)  [unwired: 4 in]
      n99 = node-c288(w160) -> (w162:T15)  [unwired: 3 in]
      n100 = timed-loop {
        timing: w159 -> [_]
        timing-out: [_] -> w158
        i -> [w178]
        stop <- w177 stop-if-true
        n101 = node-c288() -> (→"SlowLoop":bool, w175:i64)  [unwired: 1 in]
        n102 = disable-structure shown="Disabled" {
          frame Disabled {
            n103 = event shown="[1] \"RecordsSelection\": Value Change" {
              selector: _ -> [_ _]
              dyn-events: _ -> [_ _]
              timeout: 0 -> [_ _]
              event Timeout {
                n104 = event-data() -> ()  [unwired: 1 in, 2 out]
              }
              event "RecordsSelection": Value Change {
                n105 = event-data() -> ()  [unwired: 1 in, 5 out]
                n106 = local read "RecordsSelection"() -> (w189:string)
                n107 = local read "DatabaseUDL"() -> (w181:path)
                n108 = Open Application Reference(10:u16 3362 ("port number or service name (3363)"), 11:"192.168.0.1" ("machine name (\"\":  open local reference)")) -> (3:w186:refnum<vi>)  [unwired: 2 in, 1 out]
                n109 = Open VI Reference(type specifier VI Refnum (for type only)=refnum<vi> refnum, application reference (local)=w186, vi path=path "E:/Code/PID/SubVIs/UpdateDatabase.vi") -> (vi reference=w183:refnum<vi>)  [unwired: 3 in, 1 out]
                n110 = call-by-ref "?"(reference=w183, "RecordsSelection"=w189, "CallType"=enum16{"Initialize", "Save", "Load"}."Load", "DatabaseUDL"=w181) -> ("DatabaseOut"=w190:T2)  [unwired: 2 in, 4 out]
                n111 = local write "Database"(w190) -> ()
              }
            }
          }
          frame Enabled {
          }
        }
        n112 = local read "EncPos"() -> (w166:cluster{"[0]":dbl, "[1]":dbl, "[2]":dbl})
        n113 = local read "DesiredPos"() -> (w168:dbl[])
        n114 = Cluster To Array(cluster=w166) -> (array=w167:dbl[])
        n115 = Subtract(x=w167, y=w168) -> (x-y=w169:dbl[])
        n116 = feedback #1() -> (w163:u32)  [unwired: 1 in]
        n117 = Absolute Value(x=w169) -> (abs(x)=w164:dbl[])
        n118 = Less?(x=w164, y=1) -> (x < y?=w171:bool[])
        n119 = Divide(x=w175, y=i64 1000) -> (x/y=→"LoopPeriod":dbl)
        n120 = Boolean Array To Number(Boolean array=w171) -> (number=w165:u32)
        n121 = feedback-in #1(w165) -> ()
        n122 = Not Equal?(x=w165, y=w163) -> (x != y?=w172:bool)
        n123 = case shown="True" w172 {
          tunnel: w165 -> [_ w191]
          frame False {
          }
          frame True {
            n124 = case shown="0, Default" w191 {
              tunnel: [cluster{u32, u32} {11372, 11372} cluster{u32, u32} {2269951, 2269951} cluster{u32, u32} {11372, 11372} cluster{u32, u32} {2269951, 2269951} cluster{u32, u32} {11372, 11372} cluster{u32, u32} {2269951, 2269951} cluster{u32, u32} {11372, 11372} cluster{u32, u32} {2269951, 2269951}] -> w194
              tunnel: [cluster{u32, u32} {7405568, 7405568} cluster{u32, u32} {7405568, 7405568} cluster{u32, u32} {7405568, 7405568} cluster{u32, u32} {7405568, 7405568} cluster{u32, u32} {16717591, 16717591} cluster{u32, u32} {16717591, 16717591} cluster{u32, u32} {16717591, 16717591} cluster{u32, u32} {16717591, 16717591}] -> w193
              tunnel: [cluster{u32, u32} {2113536, 2113536} cluster{u32, u32} {2113536, 2113536} cluster{u32, u32} {8453888, 8453888} cluster{u32, u32} {8453888, 8453888} cluster{u32, u32} {2113536, 2113536} cluster{u32, u32} {2113536, 2113536} cluster{u32, u32} {8453888, 8453888} cluster{u32, u32} {8453888, 8453888}] -> w192
              frame 0, Default {
              }
              frame 1 {
              }
              frame 2 {
              }
              frame 3 {
              }
              frame 4 {
              }
              frame 5 {
              }
              frame 6 {
              }
              frame 7 {
              }
            }
            n125 = property on="Middle" class="Slide (strict)"("Slider Colors"=w192) -> ()  [unwired: 2 in, 2 out]
            n126 = property on="Index" class="Slide (strict)"("Slider Colors"=w194) -> ()  [unwired: 2 in, 2 out]
            n127 = property on="Thumb" class="Slide (strict)"("Slider Colors"=w193) -> ()  [unwired: 2 in, 2 out]
          }
        }
        n128 = local read "Current State"() -> (w176:T3)
        n129 = case shown="\"Acquire Response\"" w176 {
          frame "Initialize", Default {
            n130 = local read "LoopCount"() -> (w221:u64)
            n131 = local read "InitialForce"() -> (w224:dbl[])
            n132 = call "LoopComp.vi"("LoopCount"=w221, "Instance"=0, "Mode"=enum16{"Reset", "Run"}."Reset") -> ()  [unwired: 3 in, 2 out]
            n133 = local write "Current State"(T3."Acquire Start" ("Current State")) -> ()
            n134 = local write "Finalize"(enum16{"Reward", "Cerebus", "Reset"}."Reward" ("Finalize")) -> ()
            n135 = local write "SetPoint"(w224) -> ()
            n136 = call "RunOnce.vi"("Instance"=0, "Mode"=enum16{"Reset", "Run"}."Reset") -> ()  [unwired: 1 out]
          }
          frame "Acquire Start" {
            n137 = local read "EncPos"() -> (w232:cluster{"[0]":dbl, "[1]":dbl, "[2]":dbl})
            n138 = local read "DesiredPos"() -> (w227:dbl[])
            n139 = Cluster To Array(cluster=w232) -> (array=w229:dbl[])
            n140 = Subtract(x=w229, y=w227) -> (x-y=w231:dbl[])
            n141 = Absolute Value(x=w231) -> (abs(x)=w233:dbl[])
            n142 = Less?(x=w233, y=1) -> (x < y?=w230:bool[])
            n143 = And Array Elements(Boolean array=w230) -> (logical AND=w228:bool)
            n144 = case shown="True" w228 {
              frame False {
                n145 = local read "LoopCount"() -> (w235:u64)
                n146 = call "LoopComp.vi"("LoopCount"=w235, "Instance"=0, "Mode"=enum16{"Reset", "Run"}."Reset") -> ()  [unwired: 3 in, 2 out]
              }
              frame True {
                n147 = local read "Timing"() -> (w239:T1)
                n148 = local read "LoopPeriod"() -> (w245:u64)
                n149 = local read "LoopCount"() -> (w242:u64)
                n150 = Unbundle By Name(w239) -> ("ASD"=w238:u64)
                n151 = call "LoopComp.vi"("RandTime"=u64 200, "LoopPeriod"=w245, "SetTime"=w238, "LoopCount"=w242, "Instance"=0, "Mode"=enum16{"Reset", "Run"}."Run") -> ("Outcome"=w240:enum16{"TimeIn", "TimeOut"})  [unwired: 1 out]
                n152 = case shown="\"TimeOut\"" w240 {
                  frame "TimeIn", Default {
                  }
                  frame "TimeOut" {
                    n153 = local read "RandFinger"() -> (w251:bool)
                    n154 = local read "RandForce"() -> (w248:bool)
                    n155 = case shown="True" w251 {
                      frame False {
                      }
                      frame True {
                        n156 = Random Number (0-1)() -> (number: 0 to 1=w267:dbl)
                        n157 = Multiply(x=w267, y=3.0) -> (x*y=w265:dbl)
                        n158 = Round Toward -Infinity(1:w265) -> (0:w266:dbl)
                        n159 = local write "TrialType"(w266) -> ()
                      }
                    }
                    n160 = case shown="True" w248 {
                      frame False {
                      }
                      frame True {
                        n161 = local read "MaxForce"() -> (w256:dbl)
                        n162 = Random Number (0-1)() -> (number: 0 to 1=w258:dbl)
                        n163 = Random Number (0-1)() -> (number: 0 to 1=w264:dbl)
                        n164 = Random Number (0-1)() -> (number: 0 to 1=w259:dbl)
                        n165 = Multiply(x=w264, y=w256) -> (x*y=w263:dbl)
                        n166 = Multiply(x=w258, y=w256) -> (x*y=w257:dbl)
                        n167 = Multiply(x=w259, y=w256) -> (x*y=w260:dbl)
                        n168 = Round Toward -Infinity(1:w263) -> (0:w261:dbl)
                        n169 = Round Toward -Infinity(1:w257) -> (0:w254:dbl)
                        n170 = Round Toward -Infinity(1:w260) -> (0:w255:dbl)
                        n171 = Build Array(w261, w255, w254) -> (w262:dbl[])
                        n172 = local write "RampGain"(w262) -> ()
                      }
                    }
                    n173 = local read "LoopCount"() -> (w250:u64)
                    n174 = local read "EncPos"() -> (w252:cluster{"[0]":dbl, "[1]":dbl, "[2]":dbl})
                    n175 = local write "EncStartPos"(w252) -> ()
                    n176 = local write "Current State"(T3."Acquire Response" ("Current State")) -> ()
                    n177 = call "Ramp.vi"("Mode"=enum16{"Run", "Reset"}."Reset", "LoopCount"=w250) -> ()  [unwired: 4 in, 2 out]
                    n178 = call "SendCerebus8.vi"("String"="Start=On", "Mode"=T13."String") -> ()  [unwired: 3 in]
                  }
                }
              }
            }
          }
          frame "Acquire Response" {
            n179 = local read "EncStartPos"() -> (w274:cluster{"Index":dbl, "Middle":dbl, "Ring":dbl})
            n180 = local read "HoldRange"() -> (w269:dbl[])
            n181 = local read "EncPos"() -> (w275:cluster{"[0]":dbl, "[1]":dbl, "[2]":dbl})
            n182 = Cluster To Array(cluster=w275) -> (array=w270:dbl[])
            n183 = Cluster To Array(cluster=w274) -> (array=w273:dbl[])
            n184 = Subtract(x=w270, y=w273) -> (x-y=w272:dbl[])
            n185 = Absolute Value(x=w272) -> (abs(x)=w277:dbl[])
            n186 = Less?(x=w277, y=w269) -> (x < y?=w271:bool[])
            n187 = And Array Elements(Boolean array=w271) -> (logical AND=w276:bool)
            n188 = case shown="False" w276 {
              frame False {
                n189 = local read "InitialForce"() -> (w280:dbl[])
                n190 = local read "SetPoint"() -> (w281:dbl[])
                n191 = Greater?(x=w281, y=w280) -> (0:w279:bool[])
                n192 = And Array Elements(Boolean array=w279) -> (logical AND=w278:bool)
                n193 = case shown="False" w278 {
                  frame False {
                    n194 = call "RunOnce.vi"("Instance"=0, "Mode"=enum16{"Reset", "Run"}."Reset") -> ()  [unwired: 1 out]
                    n195 = local write "Current State"(T3."Finalize" ("Current State")) -> ()
                    n196 = local write "Outcome"("Abort" ("Outcome")) -> ()
                    n197 = local read "LoopCount"() -> (w291:u64)
                    n198 = call "LoopComp.vi"("LoopCount"=w291, "Instance"=0, "Mode"=enum16{"Reset", "Run"}."Reset") -> ()  [unwired: 3 in, 2 out]
                  }
                  frame True {
                    n199 = local read "InitialForce"() -> (w299:dbl[])
                    n200 = local read "LoopCount"() -> (w305:u64)
                    n201 = local read "LoopPeriod"() -> (w306:u64)
                    n202 = local read "LastCount"() -> (w297:u64)
                    n203 = local read "SetPoint"() -> (w300:dbl[])
                    n204 = Increment(x=w297) -> (x+1=w304:u64)
                    n205 = Divide(x=u64 500, y=w306) -> (x/y=w309:dbl)
                    n206 = Subtract(x=w300, y=w299) -> (x-y=w298:dbl[])
                    n207 = Subtract(x=w305, y=w304) -> (x-y=w296:u64)
                    n208 = Subtract(x=w296, y=w309) -> (x-y=w307:dbl)
                    n209 = Divide(x=w307, y=w309) -> (x/y=w302:dbl)
                    n210 = Absolute Value(x=w302) -> (abs(x)=w301:dbl)
                    n211 = Multiply(x=w298, y=w301) -> (x*y=w303:dbl[])
                    n212 = local write "SetPoint"(w303) -> ()
                  }
                }
                n213 = call "RunOnce.vi"("Instance"=0, "Mode"=enum16{"Reset", "Run"}."Reset") -> ()  [unwired: 1 out]
                n214 = local read "LoopCount"() -> (w286:u64)
                n215 = local write "Current State"(T3."Finalize" ("Current State")) -> ()
                n216 = local write "Outcome"("Abort" ("Outcome")) -> ()
                n217 = call "LoopComp.vi"("LoopCount"=w286, "Instance"=0, "Mode"=enum16{"Reset", "Run"}."Reset") -> ()  [unwired: 3 in, 2 out]
              }
              frame True {
                n218 = local read "Timing"() -> (w312:T1)
                n219 = local read "LoopPeriod"() -> (w321:u64)
                n220 = local read "LoopCount"() -> (w322:u64)
                n221 = Unbundle By Name(w312) -> ("RampTime"=w310:u64, "HoldTime"=w311:u64)
                n222 = local read "InitialForce"() -> (w316:dbl[])
                n223 = local read "RampGain"() -> (w317:dbl[])
                n224 = call "Ramp.vi"("LoopPeriod"=w321, "HoldTime"=w311, "RampTime"=w310, "Mode"=enum16{"Run", "Reset"}."Run", "LoopCount"=w322) -> ("Value"=w319:dbl, "Outcome"=w320:enum16{"RampUp", "Hold", "RampDown", "Finished"})  [unwired: 1 in]
                n225 = Multiply(x=w319, y=w317) -> (x*y=w318:dbl[])
                n226 = Add(x=w318, y=w316) -> (x+y=w315:dbl[])
                n227 = local read "RandFinger"() -> (w314:bool)
                n228 = case shown="\"Finished\"" w320 {
                  frame "RampUp", Default {
                    n229 = local read "LoopCount"() -> (→"LastCount":u64)
                  }
                  frame "Finished" {
                    n230 = local write "Current State"(T3."Finalize" ("Current State")) -> ()
                    n231 = local write "Outcome"("Success" ("Outcome")) -> ()
                    n232 = call "SendCerebus8.vi"("String"="Target=Acquired", "Mode"=T13."String") -> ()  [unwired: 3 in]
                    n233 = local read "LoopCount"() -> (w332:u64)
                    n234 = call "RunOnce.vi"("Instance"=0, "Mode"=enum16{"Reset", "Run"}."Reset") -> ()  [unwired: 1 out]
                    n235 = call "LoopComp.vi"("LoopCount"=w332, "Instance"=0, "Mode"=enum16{"Reset", "Run"}."Reset") -> ()  [unwired: 3 in, 2 out]
                  }
                }
                n236 = case shown="True" w314 {
                  tunnel: w315 -> [w323 w326]
                  frame False {
                    n237 = local write "SetPoint"(w323) -> ()
                  }
                  frame True {
                    n238 = local read "TrialType"() -> (w324:i32)
                    n239 = local read "SetPoint"() -> (w327:dbl[])
                    n240 = Index Array(array=w326, index=w324) -> (element=w325:dbl)
                    n241 = Replace Array Subset(array=w327, new element=w325, index=w324) -> (w328:dbl[])
                    n242 = local write "SetPoint"(w328) -> ()
                  }
                }
              }
            }
          }
          frame "Finalize" {
            n243 = local read "Finalize"() -> (w339:enum16{"Reward", "Cerebus", "Reset"})
            n244 = case shown="\"Reward\", Default" w339 {
              frame "Reward", Default {
                n245 = local read "Outcome"() -> (w340:string)
                n246 = case shown="\"Success\"" w340 {
                  frame "Abort", Default {
                    n247 = local read "Timing"() -> (w342:T1)
                    n248 = local read "LoopPeriod"() -> (w348:u64)
                    n249 = local read "LoopCount"() -> (w345:u64)
                    n250 = Unbundle By Name(w342) -> ("AbortTime"=w341:dbl)
                    n251 = call "LoopComp.vi"("RandTime"=u64 200, "LoopPeriod"=w348, "SetTime"=w341, "LoopCount"=w345, "Instance"=0, "Mode"=enum16{"Reset", "Run"}."Run") -> ("Outcome"=w344:enum16{"TimeIn", "TimeOut"})  [unwired: 1 out]
                    n252 = case shown="\"TimeIn\", Default" w344 {
                      frame "TimeIn", Default {
                        n253 = call-poly <vilib>:"DAQmx Write.vi"("task/channels in"=refnum<k21> "sound", "data"=1.0) -> ()  [unwired: 11 in, 3 out]
                      }
                      frame "TimeOut" {
                        n254 = local write "Finalize"(enum16{"Reward", "Cerebus", "Reset"}."Cerebus" ("Finalize")) -> ()
                      }
                    }
                  }
                  frame "Success" {
                    n255 = local read "Timing"() -> (w353:T1)
                    n256 = local read "LoopPeriod"() -> (w359:u64)
                    n257 = local read "LoopCount"() -> (w355:u64)
                    n258 = Unbundle By Name(w353) -> ("JuiceTime"=w352:dbl)
                    n259 = call "LoopComp.vi"("RandTime"=u64 200, "LoopPeriod"=w359, "SetTime"=w352, "LoopCount"=w355, "Instance"=0, "Mode"=enum16{"Reset", "Run"}."Run") -> ("Outcome"=w358:enum16{"TimeIn", "TimeOut"})  [unwired: 1 out]
                    n260 = case shown="\"TimeIn\", Default" w358 {
                      frame "TimeIn", Default {
                        n261 = call "RunOnce.vi"("Instance"=0, "Mode"=enum16{"Reset", "Run"}."Run") -> ("State"=w362:enum16{"RunOnce", "Finished"})
                        n262 = case shown="\"RunOnce\", Default" w362 {
                          frame "RunOnce", Default {
                            n263 = call-poly <vilib>:"DAQmx Write.vi"("task/channels in"=refnum<k21> "JuiceAndScreen", "data"=5.0) -> ()  [unwired: 11 in, 3 out]
                          }
                          frame "Finished" {
                          }
                        }
                      }
                      frame "TimeOut" {
                        n264 = local write "Finalize"(enum16{"Reward", "Cerebus", "Reset"}."Cerebus" ("Finalize")) -> ()
                        n265 = call-poly <vilib>:"DAQmx Write.vi"("task/channels in"=refnum<k21> "JuiceAndScreen", "data"=0.0) -> ()  [unwired: 11 in, 3 out]
                      }
                    }
                  }
                }
              }
              frame "Cerebus" {
                n266 = disable-structure shown="Disabled" {
                  frame Disabled {
                    # "*ExpParameter:Intensity=1.02;Duration=400;Trials=1;PageSegment=14;#\n*Stimulation:StimCount=5;Duration=10;#\n*WaitSeconds=10;#\n*JuiceStatus=ON;#"
                    n267 = local read "TrialType"() -> (w385:i32)
                    n268 = case shown="0, Default" w385 {
                      selector: w385 -> [w386 w391 w395]
                      tunnel: ["Target=Thumb;" ("Key Word") "Target=Index;" ("Key Word") "Target=Middle;" ("Key Word")] -> w381
                      tunnel: [w388 w390 w394] -> w369
                      frame 0, Default {
                        n269 = local read "DesiredPos"() -> (w389:dbl[])
                        n270 = Index Array(array=w389, index=w386) -> (element=w388:dbl)
                      }
                      frame 1 {
                        n271 = local read "DesiredPos"() -> (w392:dbl[])
                        n272 = Index Array(array=w392, index=w391) -> (element=w390:dbl)
                      }
                      frame 2 {
                        n273 = local read "DesiredPos"() -> (w396:dbl[])
                        n274 = Index Array(array=w396, index=w395) -> (element=w394:dbl)
                      }
                    }
                    n275 = local read "TrialCount"() -> (w373:i32)
                    n276 = local read item#-1() -> (w370)
                    n277 = local read item#-1() -> (w372)
                    n278 = call "VariablesToString.vi"("Value"=w369, "Key Word"="FingerThreshold") -> ("Concatenated String"=w379:string)
                    n279 = call "VariablesToString.vi"("Value"=w370, "Key Word"="StartDuration") -> ("Concatenated String"=w377:string)
                    n280 = call "VariablesToString.vi"("Value"=w372, "Key Word"="ResponseDuration") -> ("Concatenated String"=w376:string)
                    n281 = call "VariablesToString.vi"("Value"=w373, "Key Word"="TrialCount") -> ("Concatenated String"=w375:string)
                    n282 = Concatenate Strings("TrialParameters:" ("string"), w381, w379, w377, w376, w375) -> (w383:string)
                    n283 = call "SendCerebus8.vi"("String"=w383, "Mode"=T13."String") -> ()  [unwired: 3 in]
                  }
                  frame Enabled {
                  }
                }
                n284 = local write "Finalize"(enum16{"Reward", "Cerebus", "Reset"}."Reset" ("Finalize")) -> ()
              }
              frame "Reset" {
                n285 = local read "TrialCount"() -> (w400:i32)
                n286 = local write "Outcome"("--" ("Outcome")) -> ()
                n287 = local write "Current State"(T3."Initialize" ("Current State")) -> ()
                n288 = Increment(x=w400) -> (x+1=w399:i32)
                n289 = local write "TrialCount"(w399) -> ()
              }
            }
          }
        }
        n290 = local write "LoopCount"(w178) -> ()
        n291 = local read "Stop"() -> (w177:bool)
        n292 = node-c288() -> ()  [unwired: 1 in, 1 out]
      }
      n293 = timed-loop {
        timing: w162 -> [_]
        timing-out: [_] -> w161
        stop <- w454 stop-if-true
        n294 = node-c288() -> (w456:bool, w455:i64, w438:i64)  [unwired: 1 in]
        n295 = call-poly <vilib>:"DAQmx Read.vi"("task/channels in"=refnum<k21> "PositionInA") -> ("data"=w417:dbl)  [unwired: 12 in, 2 out]
        n296 = call-poly <vilib>:"DAQmx Read.vi"("task/channels in"=refnum<k21> "PositionInB") -> ("data"=w419:dbl)  [unwired: 12 in, 2 out]
        n297 = call-poly <vilib>:"DAQmx Read.vi"("task/channels in"=refnum<k21> "PositionInC") -> ("data"=w418:dbl)  [unwired: 12 in, 2 out]
        n298 = To Double Precision Float(number=w438) -> (double precision float=w437:dbl)
        n299 = local write "SlowLoopPID"(w456) -> ()
        n300 = local write "LoopDuration(us)"(w455) -> ()
        n301 = local write "Index"(w417) -> ()
        n302 = local write "Middle"(w419) -> ()
        n303 = local write "Thumb"(w418) -> ()
        n304 = expression code="x*1e-6"(w437) -> (w445:dbl)
        n305 = local write "LoopPeriodPID(s)"(w445) -> ()
        n306 = Build Array(w417, w419, w418) -> (w410:dbl[])
        n307 = local read "BndrsCluster"() -> (w435:T6)
        n308 = local read "PIDGains"() -> (w431:T5)
        n309 = local read "SetPoint"() -> (w436:dbl[])
        n310 = local read "EncMax"() -> (w427:dbl[])
        n311 = call "PIDBoundaries.vi"("SetPointIn"=w436, "EncPosIn"=w410, "BndrsCluster"=w435, "PIDGainsIn"=w431, "EncMax"=w427) -> ("SetPointOut"=w409:dbl[], "PIDGainsOut"=w425:T4)
        n312 = Array To Cluster(array=w410) -> (cluster=w424:cluster{"[0]":dbl, "[1]":dbl, "[2]":dbl})
        n313 = Array To Cluster(array=w409) -> (cluster=w423:T25)
        n314 = local read "LP_LoadCell(Hz)"() -> (w450:dbl)
        n315 = local write "PIDGainsOut"(w425) -> ()
        n316 = local read "LoopFreq(Hz)"() -> (w443:dbl)
        n317 = local write "SetPtOut"(w423) -> ()
        n318 = local write "EncPos"(w424) -> ()
        n319 = feedback #2() -> (w444:dbl)  [unwired: 1 in]
        n320 = feedback-in #2(w443) -> ()
        n321 = feedback #3() -> (w449:dbl)  [unwired: 1 in]
        n322 = feedback-in #3(w450) -> ()
        n323 = local read "Middle"() -> (w414:dbl)
        n324 = Not Equal?(x=w443, y=w444) -> (x != y?=w441:bool)
        n325 = local read "Index"() -> (w415:dbl)
        n326 = Not Equal?(x=w450, y=w449) -> (x != y?=w442:bool)
        n327 = Build Array(w442, w441) -> (w440:bool[])
        n328 = Build Array(w415, w414) -> (w416:dbl[])
        n329 = Or Array Elements(Boolean array=w440) -> (logical OR=w439:bool)
        n330 = case shown="True" w439 {
          tunnel: [w477 w478] -> w420
          frame False {
            n331 = local read "LP_LoadCell"() -> (w477:T7)
          }
          frame True {
            n332 = local read "LP_LoadCell(Hz)"() -> (w479:dbl)
            n333 = local read "LoopFreq(Hz)"() -> (w480:dbl)
            n334 = call <vilib>:"DFD Butterworth Design.vi"("fs [Hz]"=w480, "filter type"=T18."Lowpass", "low cutoff freq [Hz]"=w479) -> ("filter out"=w478:T7)  [unwired: 7 in, 1 out]
            "LP_LoadCell" <- w478
          }
        }
        n335 = call-poly <vilib>:"DAQmx Write.vi"("task/channels in"=refnum<k21> "PosOutIM", "data"=w416) -> ()  [unwired: 11 in, 3 out]
        n336 = call-poly <vilib>:"DAQmx Read.vi"("task/channels in"=refnum<k21> "ForceInABC") -> ("data"=w430:dbl[])  [unwired: 12 in, 2 out]
        n337 = local read "Thumb"() -> (w413:dbl)
        n338 = call-poly <vilib>:"DAQmx Write.vi"("task/channels in"=refnum<k21> "PosOutT", "data"=w413) -> ()  [unwired: 11 in, 3 out]
        n339 = call-poly <vilib>:"DFD Filtering.vi"("filter"=w420, "signal in"=w430) -> ("signal out"=w408:dbl[])  [unwired: 2 in, 7 out]
        n340 = Array To Cluster(array=w408) -> (cluster=w422:T26)
        n341 = local write "LoadCell"(w422) -> ()
        n342 = call "PIDDirection.vi"("LoadCellIn"=w408, "SetPointIn"=w409) -> ("MotorDirOut"=w446:bool[])
        n343 = Negate(x="PIDLimit") -> (-x=w468:dbl)
        n344 = Negate(x="PIDLimit") -> (-x=w465:dbl)
        n345 = Negate(x="PIDLimit") -> (-x=w464:dbl)
        n346 = local read "LoopPeriodPID(s)"() -> (w452:dbl)
        n347 = local read "Linearity"() -> (w429:dbl)
        n348 = Bundle("PIDLimit"="PIDLimit", w468) -> (w463:cluster{"PIDLimit":dbl, dbl})  [unwired: 1 in]
        n349 = Bundle("PIDLimit"="PIDLimit", w465) -> (w462:cluster{"PIDLimit":dbl, dbl})  [unwired: 1 in]
        n350 = Bundle("PIDLimit"="PIDLimit", w464) -> (w461:cluster{"PIDLimit":dbl, dbl})  [unwired: 1 in]
        n351 = local write "MotorDir"(w446) -> ()
        n352 = Build Array(w429, w429, w429) -> (w428:dbl[])
        n353 = Build Array(w463, w462, w461) -> (w453:cluster{"PIDLimit":dbl, dbl}[])
        n354 = call-poly <vilib>:"DAQmx Write.vi"("task/channels in"=refnum<k21> "MotorDirABC", "data"=w446) -> ()  [unwired: 11 in, 3 out]
        n355 = call-poly <vilib>:"PID Advanced.vi"("setpoint"=w409, "output range"=w453, "process variable"=w408, "PID gains"=w425, "dt (s)"=w452, "linearity"=w428) -> ("output"=w421:dbl[])  [unwired: 8 in, 1 out]
        n356 = Absolute Value(x=w421) -> (abs(x)=w451:dbl[])
        n357 = Subtract(x=1.0 ("y"), y=w451) -> (x-y=w474:dbl[])
        n358 = local read "PWMFreq(Hz)"() -> (w432:dbl)
        n359 = In Range and Coerce(upper limit=0.999, x=w474, lower limit=0.001) -> (coerced(x)=w459:dbl[])  [unwired: 1 out]
        n360 = local read "LoopFreq(Hz)"() -> (w434:dbl)
        n361 = Index Array(array=w459) -> (element #1=w426:dbl, element #2=w458:dbl, element #3=w457:dbl)  [unwired: 3 in]
        n362 = local read "PWMTaskA"() -> (w469:refnum<k21>)
        n363 = local read "PWMTaskC"() -> (w447:refnum<k21>)
        n364 = local read "PWMTaskB"() -> (w467:refnum<k21>)
        n365 = expression code="(1/x)*1e6"(w434) -> (w433:dbl)
        n366 = local read "Stop"() -> (w454:bool)
        n367 = node-c288(w433) -> ()  [unwired: 1 out]
        n368 = call-poly <vilib>:"DAQmx Write.vi"("task/channels in"=w469, "frequency"=w432, "duty cycle"=w426) -> ()  [unwired: 10 in, 3 out]
        n369 = call-poly <vilib>:"DAQmx Write.vi"("task/channels in"=w467, "frequency"=w432, "duty cycle"=w458) -> ()  [unwired: 10 in, 3 out]
        n370 = call-poly <vilib>:"DAQmx Write.vi"("task/channels in"=w447, "frequency"=w432, "duty cycle"=w457) -> ()  [unwired: 10 in, 3 out]
      }
      n371 = node-c288(w161) -> ()  [unwired: 1 out]
      n372 = node-c288(w158) -> ()  [unwired: 1 out]
    }
    frame #3 {
      n373 = local read "PWMTaskA"() -> (w509:refnum<k21>)
      n374 = local read "PWMTaskB"() -> (w507:refnum<k21>)
      n375 = local read "PWMTaskC"() -> (w501:refnum<k21>)
      n376 = call <vilib>:"DAQmx Stop Task.vi"("task/channels in"=refnum<k21> "sound") -> ("error out"=w496:errorcluster)  [unwired: 13 in, 1 out]
      n377 = call <vilib>:"DAQmx Stop Task.vi"("task/channels in"=refnum<k21> "ForceInABC") -> ("error out"=w512:errorcluster)  [unwired: 13 in, 1 out]
      n378 = call <vilib>:"DAQmx Stop Task.vi"("task/channels in"=refnum<k21> "MotorDirABC") -> ("error out"=w513:errorcluster)  [unwired: 13 in, 1 out]
      n379 = call <vilib>:"DAQmx Clear Task.vi"("task in"=w509) -> ("error out"=w514:errorcluster)  [unwired: 14 in]
      n380 = call <vilib>:"DAQmx Clear Task.vi"("task in"=w507) -> ("error out"=w506:errorcluster)  [unwired: 14 in]
      n381 = call <vilib>:"DAQmx Clear Task.vi"("task in"=w501) -> ("error out"=w502:errorcluster)  [unwired: 14 in]
      n382 = call <vilib>:"DAQmx Stop Task.vi"("task/channels in"=refnum<k21> "PositionInA") -> ("error out"=w515:errorcluster)  [unwired: 13 in, 1 out]
      n383 = call <vilib>:"DAQmx Stop Task.vi"("task/channels in"=refnum<k21> "PositionInB") -> ("error out"=w504:errorcluster)  [unwired: 13 in, 1 out]
      n384 = call <vilib>:"DAQmx Stop Task.vi"("task/channels in"=refnum<k21> "PositionInC") -> ("error out"=w500:errorcluster)  [unwired: 13 in, 1 out]
      n385 = call <vilib>:"DAQmx Stop Task.vi"("task/channels in"=refnum<k21> "PosOutT" ("task")) -> ("error out"=w497:errorcluster)  [unwired: 13 in, 1 out]
      n386 = call <vilib>:"DAQmx Stop Task.vi"("task/channels in"=refnum<k21> "PosOutIM") -> ("error out"=w498:errorcluster)  [unwired: 13 in, 1 out]
      n387 = local write "Stop"(FALSE ("stop")) -> ()
      n388 = call <vilib>:"General Error Handler.vi"("error in (no error)"=w496) -> ()  [unwired: 10 in, 5 out]
      n389 = call <vilib>:"General Error Handler.vi"("error in (no error)"=w512) -> ()  [unwired: 10 in, 5 out]
      n390 = call <vilib>:"General Error Handler.vi"("error in (no error)"=w513) -> ()  [unwired: 10 in, 5 out]
      n391 = call <vilib>:"General Error Handler.vi"("error in (no error)"=w514) -> ()  [unwired: 10 in, 5 out]
      n392 = call <vilib>:"General Error Handler.vi"("error in (no error)"=w506) -> ()  [unwired: 10 in, 5 out]
      n393 = call <vilib>:"General Error Handler.vi"("error in (no error)"=w502) -> ()  [unwired: 10 in, 5 out]
      n394 = call <vilib>:"General Error Handler.vi"("error in (no error)"=w515) -> ()  [unwired: 10 in, 5 out]
      n395 = call <vilib>:"General Error Handler.vi"("error in (no error)"=w504) -> ()  [unwired: 10 in, 5 out]
      n396 = call <vilib>:"General Error Handler.vi"("error in (no error)"=w500) -> ()  [unwired: 10 in, 5 out]
      n397 = call <vilib>:"General Error Handler.vi"("error in (no error)"=w497) -> ()  [unwired: 10 in, 5 out]
      n398 = call <vilib>:"General Error Handler.vi"("error in (no error)"=w498) -> ()  [unwired: 10 in, 5 out]
      n399 = stacked-sequence {
        frame #0 {
          n400 = One Button Dialog(message="Make sure database is filled out!") -> (true=w516:bool)  [unwired: 1 in]
          n401 = case shown="True" w516 {
            frame False {
            }
            frame True {
              n402 = local read "DataFolder"() -> (w528:string)
              n403 = local read "StartTime"() -> (w529:timestamp)
              n404 = local read "TaskType"() -> (w527:string)
              n405 = local read "Database"() -> (w530:T2)
              n406 = Bundle By Name(cluster=w530, "ExperimentDate"=w529, "CerebusFolder"=w528, "TaskType"=w527) -> (w518:T2)
              n407 = local read "DatabaseUDL"() -> (w519:path)
              n408 = Open Application Reference(10:u16 3362 ("port number or service name (3363)"), 11:"192.168.0.1" ("machine name (\"\":  open local reference)")) -> (3:w524:refnum<vi>)  [unwired: 2 in, 1 out]
              n409 = Open VI Reference(type specifier VI Refnum (for type only)=refnum<vi> refnum, application reference (local)=w524, vi path=path "D:/Code/PID/SubVIs/UpdateDatabase.vi") -> (vi reference=w521:refnum<vi>)  [unwired: 3 in, 1 out]
              n410 = local write "Database"(w518) -> ()
              n411 = call "SendDatabase2Cerebus.vi"("Database"=w518) -> ()  [unwired: 1 out]
              n412 = call-by-ref "?"(reference=w521, "DatabaseIn"=w518, "CallType"=enum16{"Initialize", "Save", "Load"}."Save", "DatabaseUDL"=w519) -> ()  [unwired: 2 in, 5 out]
            }
          }
        }
        frame #1 {
          n413 = Open Application Reference(10:u16 3362 ("port number or service name (3363)"), 11:"192.168.0.1" ("machine name (\"\":  open local reference)")) -> (3:w536:refnum<vi>)  [unwired: 2 in, 1 out]
          n414 = Open VI Reference(type specifier VI Refnum (for type only)=refnum<vi> refnum, application reference (local)=w536, vi path=path "E:/Code/PID/SubVIs/AutoCentral.vi") -> (vi reference=w533:refnum<vi>)  [unwired: 3 in, 1 out]
          n415 = call-by-ref "?"(reference=w533, "Mode"=T14."StopRecording") -> ("Recording?"=w531:bool)  [unwired: 3 in, 4 out]
          n416 = local write "Recording"(w531) -> ()
        }
        frame #2 {
          n417 = property class="App"() -> ("Disp.AllMonitors"=w546:T19)  [unwired: 2 in, 2 out]
          n418 = Array To Cluster(array=w546) -> (cluster=w545:T20)
          n419 = Unbundle By Name(w545) -> ("Disp.AllMonitors[0].Bounds.Right"=w541:i16, "Disp.AllMonitors[0].Bounds.Bottom"=w540:i16)
          n420 = property class="VI"() -> ("Front Panel.WinBounds"=w544:T23)  [unwired: 2 in, 2 out]
          n421 = Bundle By Name(cluster=w544, "left"=i16 65, "top"=i16 0, "right"=w541, "bottom"=w540) -> (w539:T23)
          n422 = property class="VI"("Front Panel.WinBounds"=w539) -> ()  [unwired: 2 in, 2 out]
        }
        frame #3 {
          n423 = call "SendCerebus32.vi"("Mode"=T13."Close") -> ()  [unwired: 4 in]
        }
      }
    }
  }
  n424 = local read "RecordsSelection"() -> (w3:string)
  n425 = feedback #4() -> (w2:string)  [unwired: 1 in]
  n426 = feedback-in #4(w3) -> ()
  n427 = Equal?(x=w3, y=w2) -> (x = y?=w1:bool)
  n428 = case shown="False" w1 {
    frame False {
      n429 = local read "RecordsSelection"() -> (w550:string)
      n430 = local read "DatabaseUDL"() -> (w557:path)
      n431 = Open Application Reference(10:u16 3362 ("port number or service name (3363)"), 11:"192.168.0.1" ("machine name (\"\":  open local reference)")) -> (3:w553:refnum<vi>)  [unwired: 2 in, 1 out]
      n432 = Open VI Reference(type specifier VI Refnum (for type only)=refnum<vi> refnum, application reference (local)=w553, vi path=path "E:/Code/PID/SubVIs/UpdateDatabase.vi") -> (vi reference=w555:refnum<vi>)  [unwired: 3 in, 1 out]
      n433 = call-by-ref "?"(reference=w555, "RecordsSelection"=w550, "CallType"=enum16{"Initialize", "Save", "Load"}."Load", "DatabaseUDL"=w557) -> ("DatabaseOut"=w549:T2)  [unwired: 2 in, 4 out]
      n434 = local write "Database"(w549) -> ()
    }
    frame True {
    }
  }
